vi "ATF Storage-Loop control.vi"(7 "Action":enum16{"Init", "Write", "Read"}(ring), 8 "error in (no error)":errorcluster, 11 "Loop Control In":T1) -> (0 "error Out":errorcluster, 3 "Loop Control out":T1)   [LabVIEW 2022 SP3]
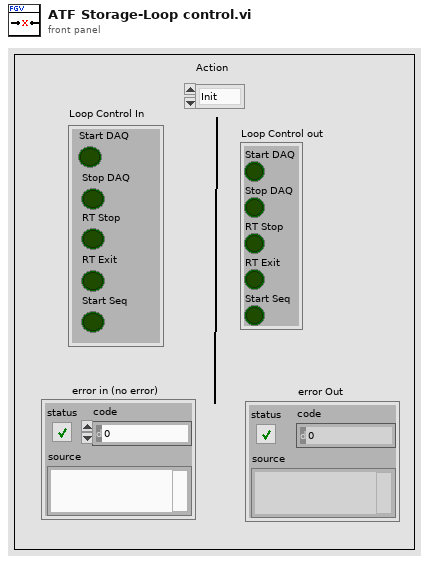
[diagram p1: front panel]
types:
  T1 = cluster{"Start DAQ":bool, "Stop DAQ":bool, "RT Stop":bool, "RT Exit":bool, "Start Seq":bool}
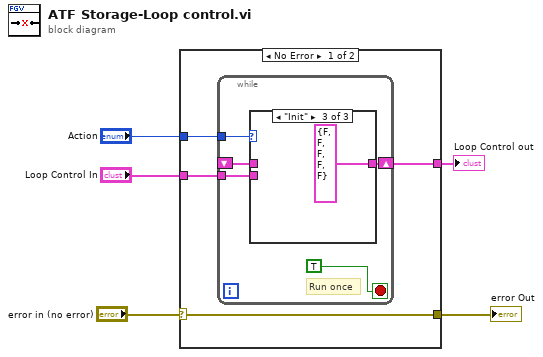
[diagram p0: block diagram]
diagram:
  n1 = case shown="No Error" "error in (no error)" {
    selector: "error in (no error)" -> [w6 _]
    tunnel: "Action" -> [w9 _]
    tunnel: "Loop Control In" -> [w8 _]
    tunnel: [w7 _] -> w1
    tunnel: [w6 _] -> w2
    frame No Error {
      n2 = while {
        tunnel: w9 -> [w13]
        tunnel: w8 -> [w12]
        shift-right: [w11] -> w7
        shift-left: _ -> [w10]
        stop <- TRUE stop-if-true
        # "Run once"
        n3 = case shown="\"Init\"" w13 {
          tunnel: w12 -> [w15 _ _]
          tunnel: [w15 w16 T1 {"Start DAQ"=FALSE, "Stop DAQ"=FALSE, "RT Stop"=FALSE, "RT Exit"=FALSE, "Start Seq"=FALSE} ("Loop Control In")] -> w11
          tunnel: w10 -> [_ w16 _]
          frame "Write" {
          }
          frame "Read", Default {
          }
          frame "Init" {
          }
        }
      }
    }
    frame Error {
    }
  }
  "error Out" <- w2
  "Loop Control out" <- w1
